vi "240124_Init-PI_C867.vi"(8 "error in (no error)":errorcluster) -> (0 "error out":errorcluster, 3 "C-867-cluster":T1)   [LabVIEW 2014]
doc: "This VI is used to initialize the XY stage (C-867).\nIt:\n- starts the communication on the USB port\n- starts to reference all axes\n- sets servo ON and validates this\n- get the current name of the axes\n- get the current positions of the stage\n- get the range of the axes"
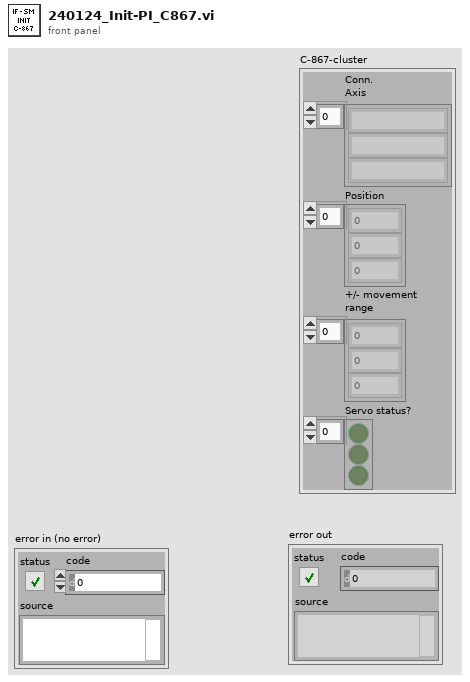
[diagram p1: front panel]
types:
  T1 = cluster{"Conn. \nAxis":string[], "Position":dbl[], "+/- movement\nrange":dbl[], "Servo status?":bool[]}
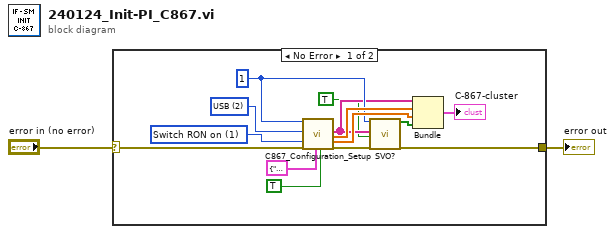
[diagram p0: block diagram]
diagram:
  n1 = case shown="No Error" "error in (no error)" {
    selector: "error in (no error)" -> [w16 w17]
    tunnel: [w8 w17] -> w1
    frame No Error {
      w13 = u16 1 items=["Default", "Switch RON on", "Switch RON off"] ("Reference mode")
      w14 = u16 2 items=["RS232", "RS232 DaisyChain", "USB"] ("Interface")
      w7 = 1 ("System no.")
      n2 = call "C867_Configuration_Setup.vi"("System no."=w7, "Interface"=w14, "Reference mode"=w13, "error in"=w16, "USB settings"=cluster{"S/N":string, "USB Search?":bool} {"S/N"="0115045905", "USB Search?"=TRUE}, "Switch servo on?"=TRUE) -> ("Conn. \nAxis"=w6:string[], "Position"=w11:dbl[], "+/- movement\nrange"=w10:dbl[], "error out"=w9:errorcluster)  [unwired: 7 in, 3 out]
      n3 = call "SVO?.vi"("System no."=w7, "Axes to query"=w6, "All axes?"=TRUE, "error in"=w9) -> ("Servo status?"=w4:bool[], "error out"=w8:errorcluster)  [unwired: 14 in]
      n4 = Bundle("Conn. \nAxis"=w6, "Position"=w11, "+/- movement\nrange"=w10, "Servo status?"=w4) -> (→"C-867-cluster":T1)  [unwired: 1 in]
    }
    frame Error {
    }
  }
  "error out" <- w1
